vi "Test of Shortcut Menu from Cluster.vi"() -> ()   [LabVIEW 2019]
uses:
  Menu From Cluster.lvlib
panel:
  out "item tag":string
  in  "String":string
  out "Item":string
  out "ItemTag":string
  out "A control or indicator":cluster{"X":dbl, "Y":dbl}[](graph)
  # "Run this program, then right-click this control and experiment changing Options"
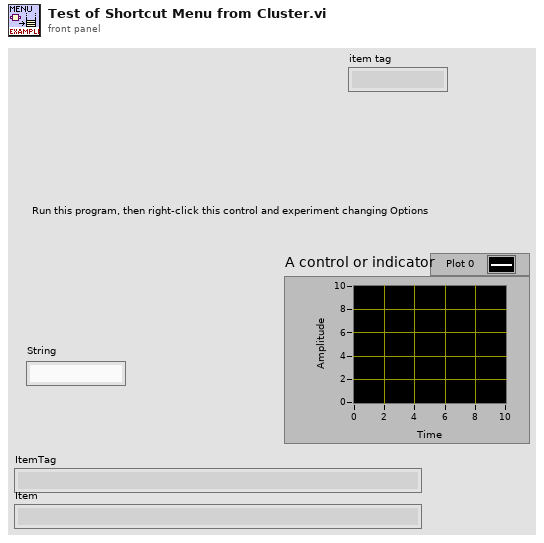
[diagram p1: front panel]
types:
  T1 = cluster{"B Enum":enum16{"Item1", "Item2", "Item3"}, "B Boolean":bool, "Options2":cluster{"Another Enum":enum16{"Item1", "Item2", "Item3"}, "Another boolean":bool}}
  T2 = cluster{"An Enum":enum16{"Item1", "Item2", "Item3"}, "A Boolean":bool, "Options":cluster{"Sub Enum":enum16{"Item1", "Item2", "Item3"}, "Sub Boolean":bool}}
  T3 = cluster{"Options Menu":cluster{"An Enum":enum16{"Item1", "Item2", "Item3"}, "A Boolean":bool, "Options":cluster{"Sub Enum":enum16{"Item1", "Item2", "Item3"}, "Sub Boolean":bool}}, "More Options":cluster{"B Enum":enum16{"Item1", "Item2", "Item3"}, "B Boolean":bool, "Options2":cluster{"Another Enum":enum16{"Item1", "Item2", "Item3"}, "Another boolean":bool}}}
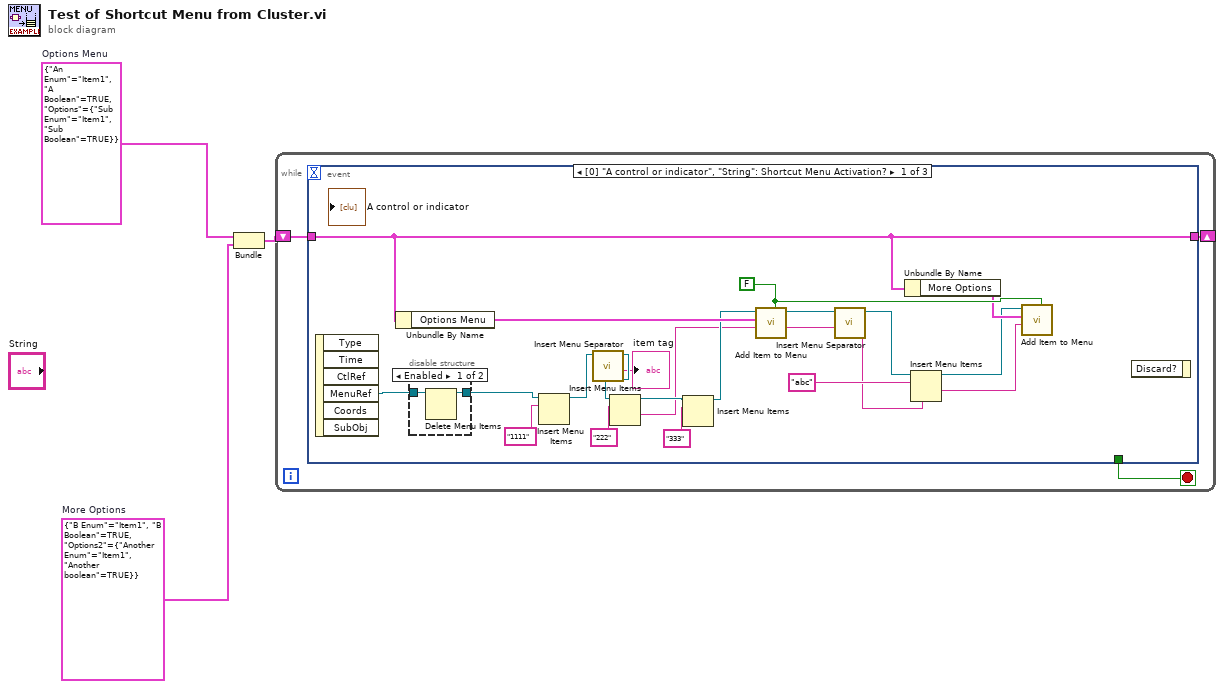
[diagram p0: block diagram]
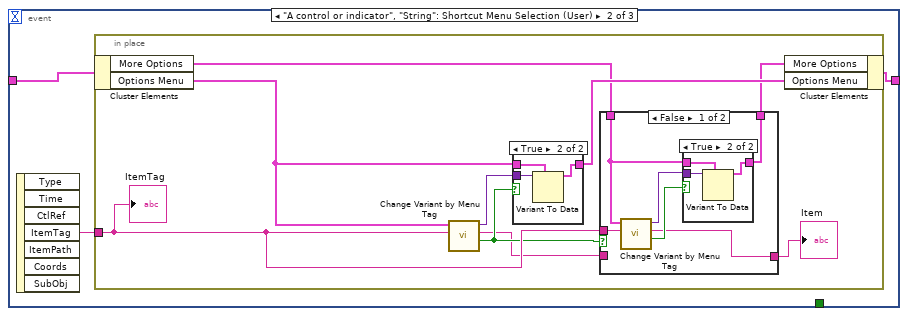
[diagram p3: hidden frame]
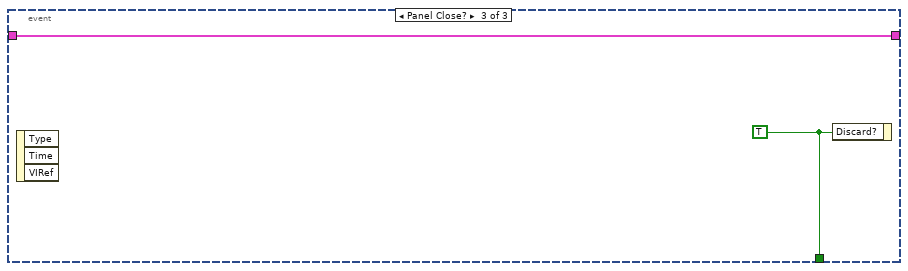
[diagram p7: hidden frame]
diagram:
  w1 = T1 {"B Enum"=enum."Item1", "B Boolean"=TRUE, "Options2"={"Another Enum"=enum."Item1", "Another boolean"=TRUE}}  # More Options
  w2 = T2 {"An Enum"=enum."Item1", "A Boolean"=TRUE, "Options"={"Sub Enum"=enum."Item1", "Sub Boolean"=TRUE}}  # Options Menu
  n1 = Bundle("Options Menu"=w2, "More Options"=w1) -> (w3:T3)  [unwired: 1 in]
  n2 = while {
    shift-right: [w5] -> _
    shift-left: w3 -> [w6]
    stop <- w4 stop-if-true
    n3 = event shown="[0] \"A control or indicator\", \"String\": Shortcut Menu Activation?" {
      selector: _ -> [_ _ _]
      dyn-events: _ -> [_ _ _]
      timeout: _ -> [_ _ _]
      tunnel: w6 -> [w26 w34 w61]
      tunnel: [w26 w33 w61] -> w5
      tunnel: [_ _ w60] -> w4
      event "A control or indicator", "String": Shortcut Menu Activation? {
        w19 = FALSE ("Create Submenu if a Cluster")
        n4 = event-data() -> ("MenuRef"=w28:refnum<k9>)  [unwired: 1 in, 5 out]
        n5 = Unbundle By Name(w26) -> ("Options Menu"=w27:T2)
        n6 = disable-structure shown="Enabled" {
          disable-tunnel: w28 -> [w30 w31]
          disable-tunnel: [w29 w31] -> w24
          frame Enabled {
            n7 = Delete Menu Items(9:w30) -> (3:w29:refnum<k9>)  [unwired: 3 in, 1 out]
          }
          frame Disabled {
          }
        }
        n8 = Insert Menu Items(8:"1111", 9:w24) -> (3:w15:refnum<k9>)  [unwired: 4 in, 2 out]
        n9 = call "Insert Menu Separator.vi"("Menu in"=w15) -> ("item tag"=→"item tag":string, "Menu out"=w14:refnum<k9>)  [unwired: 9 in]
        n10 = Insert Menu Items(8:"222", 9:w14) -> (1:w7:string, 3:w21:refnum<k9>)  [unwired: 4 in, 1 out]
        n11 = Insert Menu Items(8:"333", 9:w21) -> (3:w20:refnum<k9>)  [unwired: 4 in, 2 out]
        n12 = call "Add Item to Menu.vi"("Create Submenu if a Cluster"=w19, "after item"=w7, "Item(s) to Add"=w27, "menu reference"=w20) -> ("last root-level item"=w10:string, "menu reference out"=w13:refnum<k9>)  [unwired: 5 in, 1 out]
        n13 = call "Insert Menu Separator.vi"("after item"=w10, "Menu in"=w13) -> ("item tag"=w11:string, "Menu out"=w12:refnum<k9>)  [unwired: 8 in]
        n14 = Unbundle By Name(w26) -> ("More Options"=w17:T1)
        n15 = Insert Menu Items(4:w11, 8:"abc", 9:w12) -> (1:w9:string, 3:w16:refnum<k9>)  [unwired: 3 in, 1 out]
        n16 = call "Add Item to Menu.vi"("Create Submenu if a Cluster"=w19, "after item"=w9, "Item(s) to Add"=w17, "menu reference"=w16) -> ()  [unwired: 5 in, 3 out]
        n17 = event-data() -> ()  [unwired: 2 in, 1 out]
      }
      event "A control or indicator", "String": Shortcut Menu Selection (User) {
        n18 = event-data() -> ("ItemTag"=w32:string)  [unwired: 1 in, 6 out]
        n19 = in-place {
          in-place-border: w32 -> [w38]
          n20 = in-place-cluster #1(w34) -> ("More Options"=w40:T1, "Options Menu"=w42:T2)
          n21 = call "Change Variant by Menu Tag.vi"("tag"=w38, "Cluster"=w42) -> ("Cluster Changed"=w37:bool, "Item"=w36:string, "VCluster out"=w41:variant)  [unwired: 6 in, 1 out]
          n22 = case shown="True" w37 {
            tunnel: w41 -> [_ w59]
            tunnel: [w56 w58] -> w43
            tunnel: w42 -> [w56 w57]
            frame False {
            }
            frame True {
              n23 = Variant To Data(type=w57, Variant=w59) -> (data=w58:T2)  [unwired: 1 in, 1 out]
            }
          }
          n24 = case shown="False" w37 {
            tunnel: w40 -> [w47 w55]
            tunnel: [w46 w55] -> w39
            tunnel: w38 -> [w45 _]
            tunnel: [w44 w54] -> w35
            tunnel: w36 -> [_ w54]
            frame False {
              n25 = call "Change Variant by Menu Tag.vi"("tag"=w45, "Cluster"=w47) -> ("Cluster Changed"=w48:bool, "Item"=w44:string, "VCluster out"=w49:variant)  [unwired: 6 in, 1 out]
              n26 = case shown="True" w48 {
                tunnel: w49 -> [_ w53]
                tunnel: [w50 w52] -> w46
                tunnel: w47 -> [w50 w51]
                frame False {
                }
                frame True {
                  n27 = Variant To Data(type=w51, Variant=w53) -> (data=w52:T1)  [unwired: 1 in, 1 out]
                }
              }
            }
            frame True {
            }
          }
          "Item" <- w35
          n28 = in-place-cluster #1("More Options"=w39, "Options Menu"=w43) -> (w33:T3)
          "ItemTag" <- w38
        }
      }
      event Panel Close? {
        w60 = TRUE
        n29 = event-data() -> ()  [unwired: 1 in, 3 out]
        n30 = event-data("Discard?"=w60) -> ()  [unwired: 1 in, 1 out]
      }
    }
  }
